vi "Get_Styles.vi"   [LabVIEW 2025]
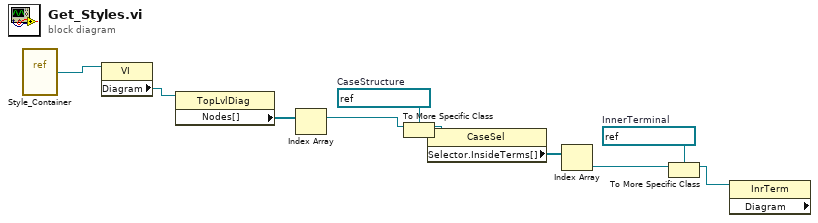
[diagram p0: block diagram]
diagram:
  w4 = refnum<vi> refnum  # InnerTerminal
  w7 = refnum<vi> refnum  # CaseStructure
  n1 = vi-ref "Style_Container.vi"() -> (w10:refnum<vi>)
  n2 = property class="VI"(reference=w10) -> ("Diagram"=w9:refnum<vi>)  [unwired: 1 in, 2 out]
  n3 = property class="TopLvlDiag"(reference=w9) -> ("Nodes[]"=w8:refnum<vi>[])  [unwired: 1 in, 2 out]
  n4 = Index Array(array=w8) -> (element=w2:refnum<vi>)  [unwired: 1 in]
  n5 = To More Specific Class(target class=w7, reference=w2) -> (specific class reference=w3:refnum<vi>)  [unwired: 1 in, 1 out]
  n6 = property class="CaseSel"(reference=w3) -> ("Selector.InsideTerms[]"=w6:refnum<vi>[])  [unwired: 1 in, 2 out]
  n7 = Index Array(array=w6) -> (element=w5:refnum<vi>)  [unwired: 1 in]
  n8 = To More Specific Class(target class=w4, reference=w5) -> (specific class reference=w1:refnum<vi>)  [unwired: 1 in, 1 out]
  n9 = property class="InrTerm" props=["Diagram"](reference=w1) -> ()  [unwired: 1 in, 3 out]
